vi "Get Configuration.vi"(8 "error in (no error)":errorcluster, 11 "Statnett C37.118 DLL in":refnum<class "Statnett C37.118 DLL.lvclass">) -> (0 "error out":errorcluster, 1 "PMU Configuration":T1(array[cluster]), 2 "PDC Configuration":T2, 3 "Statnett C37.118 DLL out":refnum<class "Statnett C37.118 DLL.lvclass">, 5 "Pseudo PDC ID":i32)   [LabVIEW 2013, in "PMU Recorder Light.lvlib" / "Statnett C37.118 DLL.lvclass"]
uses:
  Statnett C37.118 DLL.lvclass
  c37118-dll/C37118-DLL.lvlib
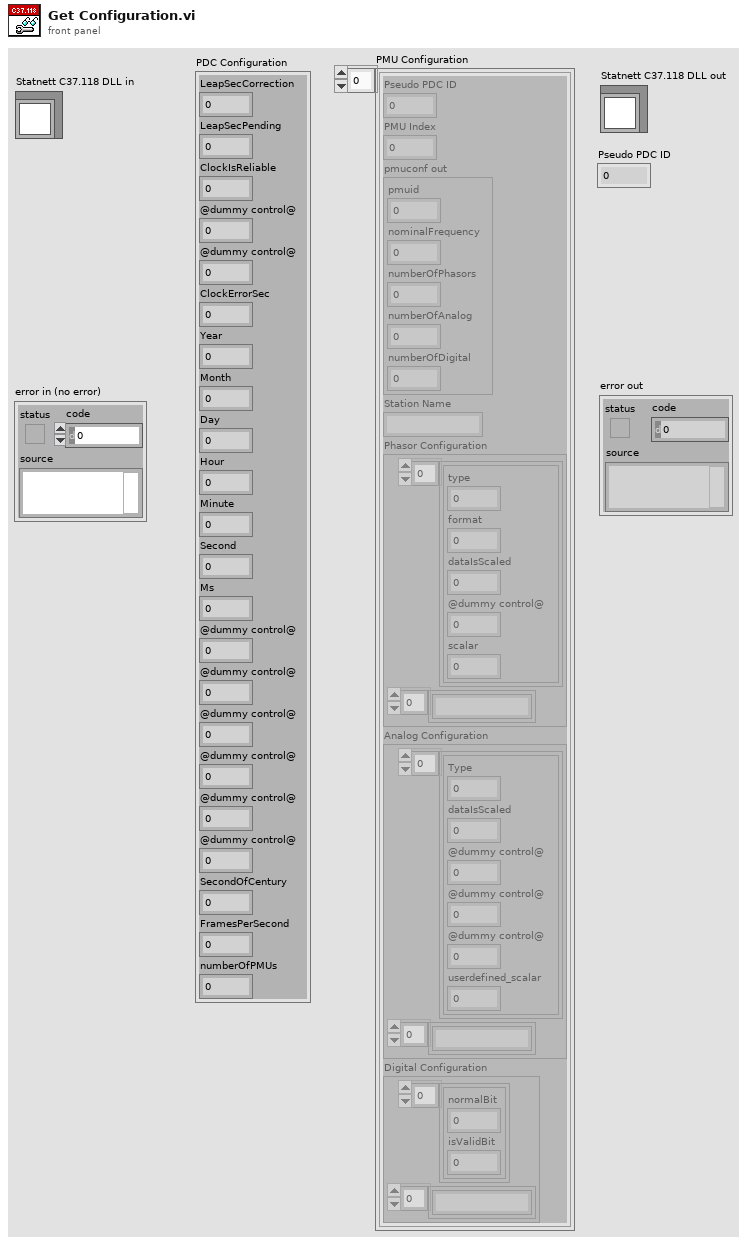
[diagram p1: front panel]
types:
  T1 = cluster{"Pseudo PDC ID":i32, "PMU Index":i32, "pmuconf out":cluster{"pmuid":i32, "nominalFrequency":sgl, "numberOfPhasors":i32, "numberOfAnalog":i32, "numberOfDigital":i32}, "Station Name":string, "Phasor Configuration":cluster{cluster{"type":u8, "format":u8, "dataIsScaled":u8, "@dummy control@":i8, "scalar":sgl}[], string[]}, "Analog Configuration":cluster{cluster{"Type":i32, "dataIsScaled":u8, "@dummy control@":i8, "@dummy control@":i8, "@dummy control@":i8, "userdefined_scalar":sgl}[], string[]}, "Digital Configuration":cluster{cluster{"normalBit":u8, "isValidBit":u8}[], string[]}}[]
  T2 = cluster{"LeapSecCorrection":i32, "LeapSecPending":u8, "ClockIsReliable":u8, "@dummy control@":i8, "@dummy control@":i8, "ClockErrorSec":sgl, "Year":i16, "Month":i16, "Day":i16, "Hour":i16, "Minute":i16, "Second":i16, "Ms":i16, "@dummy control@":i8, "@dummy control@":i8, "@dummy control@":i8, "@dummy control@":i8, "@dummy control@":i8, "@dummy control@":i8, "SecondOfCentury":dbl, "FramesPerSecond":sgl, "numberOfPMUs":i32}
  T3 = cluster{"Pseudo PDC ID":i32, "PMU Index":i32, "pmuconf out":cluster{"pmuid":i32, "nominalFrequency":sgl, "numberOfPhasors":i32, "numberOfAnalog":i32, "numberOfDigital":i32}, "Station Name":string, "Phasor Configuration":cluster{cluster{"type":u8, "format":u8, "dataIsScaled":u8, "@dummy control@":i8, "scalar":sgl}[], string[]}, "Analog Configuration":cluster{cluster{"Type":i32, "dataIsScaled":u8, "@dummy control@":i8, "@dummy control@":i8, "@dummy control@":i8, "userdefined_scalar":sgl}[], string[]}, "Digital Configuration":cluster{cluster{"normalBit":u8, "isValidBit":u8}[], string[]}}
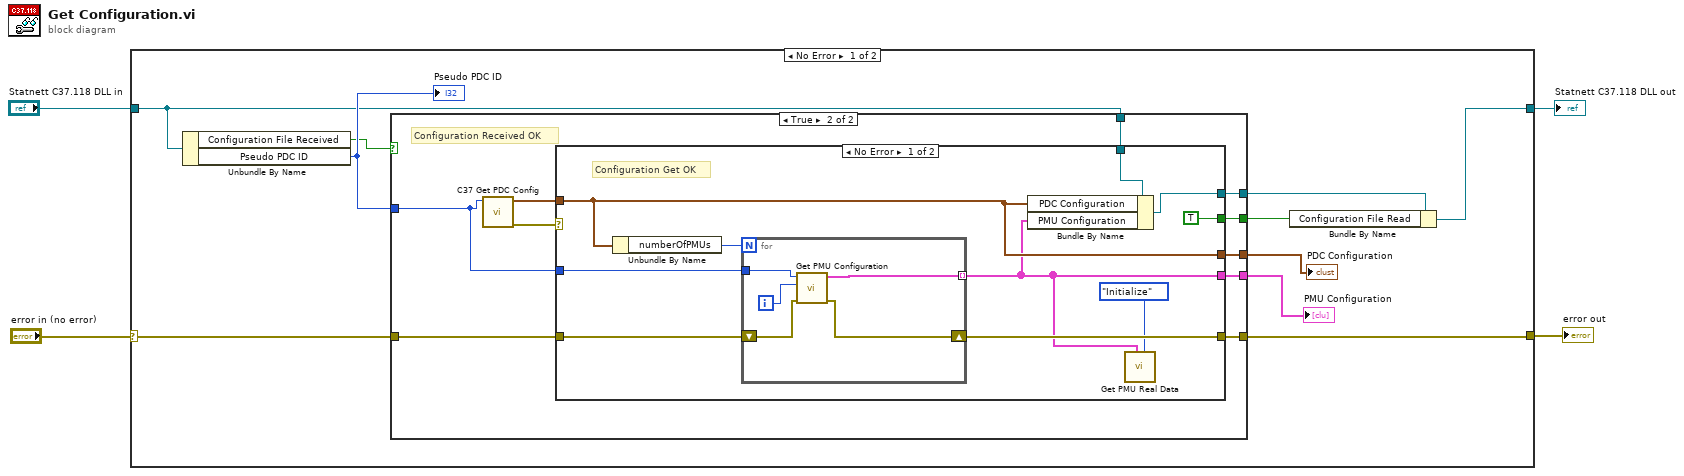
[diagram p0: block diagram]
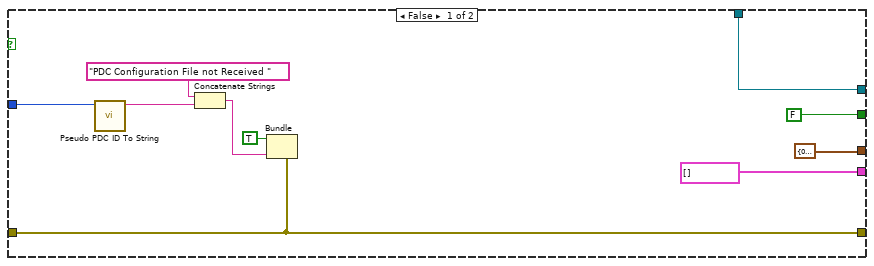
[diagram p2: hidden frame]
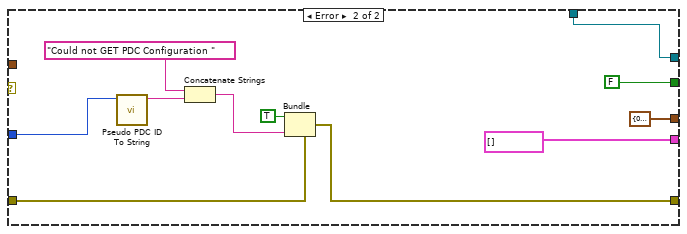
[diagram p3: hidden frame]
diagram:
  n1 = case shown="No Error" "error in (no error)" {
    selector: "error in (no error)" -> [w14 w62]
    tunnel: [w12 w62] -> w3
    tunnel: [w10 w61] -> w1
    tunnel: "Statnett C37.118 DLL in" -> [w8 w61]
    frame No Error {
      n2 = Unbundle By Name(w8) -> ("Configuration File Received"=w11:bool, "Pseudo PDC ID"=w13:i32)
      "Pseudo PDC ID" <- w13
      n3 = case shown="True" w11 {
        tunnel: w14 -> [w16 w34]
        tunnel: w13 -> [w24 w27]
        tunnel: [w16 w33] -> w12
        tunnel: [FALSE ("Configuration File Read") w32] -> w9
        tunnel: w8 -> [w18 w31]
        tunnel: [w18 w30] -> w7
        tunnel: [T2 {"LeapSecCorrection"=0, "LeapSecPending"=0, "ClockIsReliable"=0, "@dummy control@"=0, "@dummy control@"=0, "ClockErrorSec"=0.0, "Year"=0, "Month"=0, "Day"=0, "Hour"=0, "Minute"=0, "Second"=0, "Ms"=0, "@dummy control@"=0, "@dummy control@"=0, "@dummy control@"=0, "@dummy control@"=0, "@dummy control@"=0, "@dummy control@"=0, "SecondOfCentury"=0.0, "FramesPerSecond"=0.0, "numberOfPMUs"=0} ("PDC Configuration 2") w29] -> w6
        tunnel: [T1 [] ("PMU Configuration 2") w28] -> w5
        frame False {
          n4 = call "Pseudo PDC ID To String.vi"("Pseudo PDC ID"=w24) -> ("String"=w23:string)  [unwired: 10 in]
          n5 = Concatenate Strings("PDC Configuration File not Received " ("source"), w23) -> (w20:string)
          n6 = Bundle(cluster=w16, "status"=TRUE, "source"=w20) -> ()  [unwired: 1 in, 1 out]
        }
        frame True {
          # "Configuration Received OK"
          n7 = call "C37 Get PDC Config.vi"("Pseudo PDC ID"=w27) -> ("error out"=w26:errorcluster, "pdcCfg out"=w25:T2)  [unwired: 9 in]
          n8 = case shown="No Error" w26 {
            tunnel: w25 -> [w36 _]
            tunnel: w27 -> [w43 w58]
            tunnel: w34 -> [w42 w55]
            tunnel: [w41 w54] -> w33
            tunnel: [TRUE ("Configuration File Read") FALSE ("Configuration File Read")] -> w32
            tunnel: w31 -> [w38 w52]
            tunnel: [w37 w52] -> w30
            tunnel: [w36 T2 {"LeapSecCorrection"=0, "LeapSecPending"=0, "ClockIsReliable"=0, "@dummy control@"=0, "@dummy control@"=0, "ClockErrorSec"=0.0, "Year"=0, "Month"=0, "Day"=0, "Hour"=0, "Minute"=0, "Second"=0, "Ms"=0, "@dummy control@"=0, "@dummy control@"=0, "@dummy control@"=0, "@dummy control@"=0, "@dummy control@"=0, "@dummy control@"=0, "SecondOfCentury"=0.0, "FramesPerSecond"=0.0, "numberOfPMUs"=0} ("PDC Configuration 2")] -> w29
            tunnel: [w35 T1 [] ("PMU Configuration 2")] -> w28
            frame No Error {
              # "Configuration Get OK"
              n9 = Unbundle By Name(w36) -> ("numberOfPMUs"=w44:i32)
              n10 = for {
                N: w44 -> [_]
                tunnel: w43 -> [w49]
                shift-right: [w46] -> w41
                shift-left: w42 -> [w47]
                tunnel: [w45] -> w35 mode=indexing
                i -> [w48]
                n11 = call "Get PMU Configuration.vi"("error in (no error)"=w47, "PMU Index"=w48, "Pseudo PDC ID"=w49) -> ("error out"=w46:errorcluster, "PMU Configuration"=w45:T3)  [unwired: 7 in]
              }
              n12 = Bundle By Name(cluster=w38, "PDC Configuration"=w36, "PMU Configuration"=w35) -> (w37:refnum<class "Statnett C37.118 DLL.lvclass">)
              n13 = call "Get PMU Real Data.vi"("Action"=enum16{"Initialize", "Read", "Reset"}."Initialize", "PMU Configuration"=w35) -> ()  [unwired: 7 in, 3 out]
            }
            frame Error {
              n14 = call "Pseudo PDC ID To String.vi"("Pseudo PDC ID"=w58) -> ("String"=w60:string)  [unwired: 10 in]
              n15 = Concatenate Strings("Could not GET PDC Configuration " ("source"), w60) -> (w56:string)
              n16 = Bundle(cluster=w55, "status"=TRUE, "source"=w56) -> (w54:errorcluster)  [unwired: 1 in]
            }
          }
        }
      }
      "PDC Configuration" <- w6
      "PMU Configuration" <- w5
      n17 = Bundle By Name(cluster=w7, "Configuration File Read"=w9) -> (w10:refnum<class "Statnett C37.118 DLL.lvclass">)
    }
    frame Error {
    }
  }
  "error out" <- w3
  "Statnett C37.118 DLL out" <- w1
